vi "FRIC_navX_Internal_USB_ProcessingLoop.vi"(7 "Device Number":T3, 9 "Stream Type":T1=enum."AHRSAndPositioning", 10 "Serial Port":T2=enum."USB 1", 11 "Rate (4Hz-200Hz)":u8=50 min=4 max=200) -> ()   [LabVIEW 2016]
doc: "This navX VI handles the reading/writing for the navX. All of the good stuff is in here.\nTHIS VI SHOULD NOT BE CALLED BY THE USER!"
uses:
  _TypeDefs/Z900_navX_SerialStreamTypeDef.ctl
  _TypeDefs/FRIC_navX_DeviceNumbersTypeDef.ctl
  <vilib>/Rock Robotics/WPI/SerialPort/WPI_SerialPort.ctl
  _TypeDefs/FRIC_navX_I2C Process Loop TypeDef.ctl
  _TypeDefs/FRIC_navX_ProcessingLoopStatesTypeDef_I2C.ctl
  _TypeDefs/Z900_navX_DeviceTypeDef.ctl
  _TypeDefs/Z900_navX_ProtocolTypeDef.ctl
  _TypeDefs/Z900_navX_NotifyPacketTypeDef.ctl
  _TypeDefs/Z900_navX_ActionTypeDef.ctl
  <vilib>/Rock Robotics/SystemInterfaces/i2clib/i2c_bus.ctl
  _TypeDefs/Z900_navX_IntegrationControlRegisters.ctl
  <vilib>/Rock Robotics/WPI/SPI/WPI_SPIDevRef.ctl
  <vilib>/Rock Robotics/SystemInterfaces/spilib/spi_bus.ctl
  <vilib>/Rock Robotics/WPI/SerialPort/WPI_SerialPortRef.ctl
  _Device/_Internal/SERIAL/Z900_navX_SERIAL_ValidatePacketChecksum.vi
  _Device/_Internal/SERIAL/Z900_navX_SERIAL_ValidatePacketTermination.vi
  <vilib>/Rock Robotics/SystemInterfaces/Utilities/FPGA_UtilitiesRead LocalTime.vi
panel:
  in  "Tab Control":enum32{"Page 1", "Page 2"}(tab)
  in  "Halt":bool
  out "Connected 2":bool
  out "Loop Time (ms)":dbl
  out "error":errorcluster
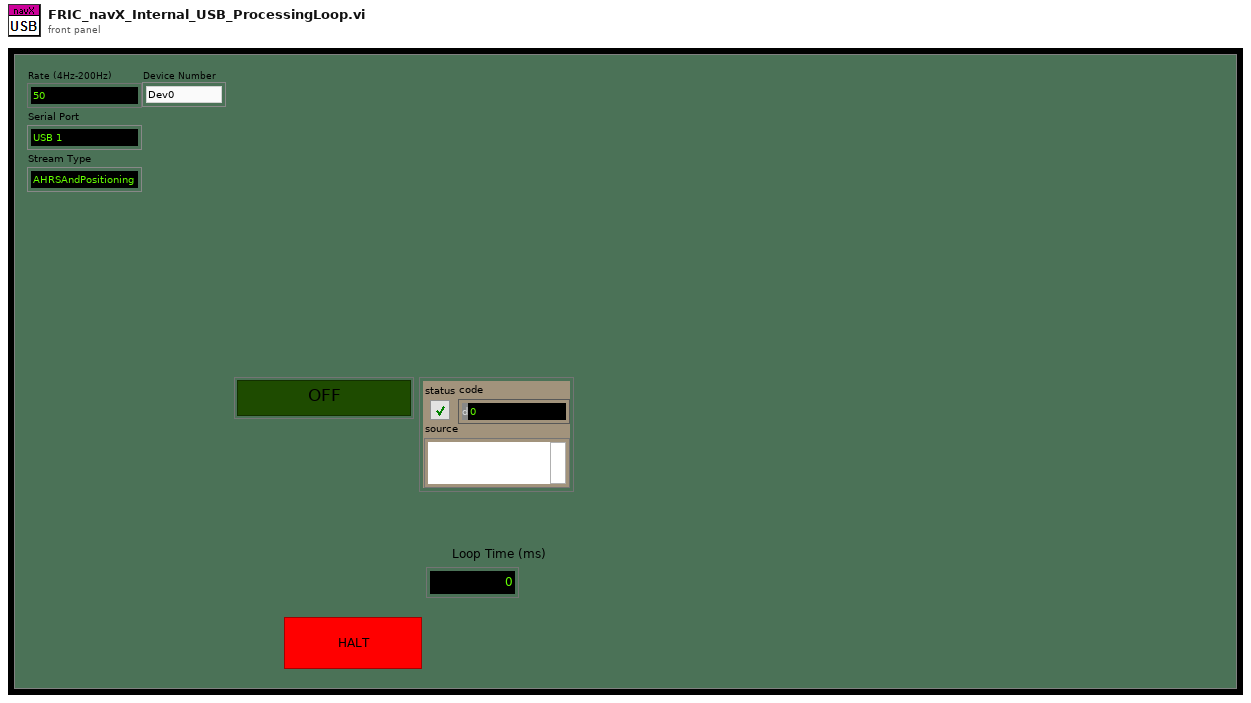
[diagram p1: front panel]
types:
  T1 = typedef "Z900_navX_SerialStreamTypeDef.ctl" = enum16{"YRPH", "Quaterinons", "Gyro/Raw", "AHRS", "AHRSAndPositioning"}
  T2 = typedef "WPI_SerialPort.ctl" = enum16{"Onboard RS-232", "MXP TTL", "USB 1", "USB 2"}
  T3 = typedef "FRIC_navX_DeviceNumbersTypeDef.ctl" = enum16{"Dev0", "Dev1", "Dev2", "Dev3", "Dev4", "Dev5", "Dev6", "Dev7", "Dev8", "Dev9", "Dev10"}
  T4 = typedef "FRIC_navX_I2C Process Loop TypeDef.ctl" = cluster{"State Array":T5[], "error":errorcluster, "FPGA Cluster":cluster{"Last Valid FPGA Time":dbl, "Error Count":i32, "Initialized":bool}, "Device Info":T6, "I2CDevRef":cluster{"DevStatus":errorcluster, "Device Address":u8, "Handle":i32, "I2C Bus":T8}, "Registry":u8[], "Command Array":T9[], "Connected?":bool, "navX Device Memory Size":i32, "notification":T10, "Memory Size Set":bool, "SPIDevRef":T12, "navX Serial Open":cluster{"Stream Type":T1, "Serial Port":T2}, "SerialPortRef":T14, "Serial Read Buffer":string, "Serial Write Buffer":string[], "Device Number":T3, "navX SPI Open":cluster{"SPI Bus":T13, "Clock Rate (Hz)":dbl}}
  T5 = typedef "FRIC_navX_ProcessingLoopStatesTypeDef_I2C.ctl" = enum16{"Process", "INI", "Check Packets Valid", "Close", "Flush Serial", "Generate Command", "Last Packet Valid", "Open", "Read", "Reset Serial", "Set Termination Char", "Update AE", "Wait", "Write", "Exit"}
  T6 = typedef "Z900_navX_DeviceTypeDef.ctl" = cluster{"Interface":cluster{"Protocol":T7, "Update Rate (4Hz-200Hz)":u8, "navX Open TypeDef":variant}, "Notify Packet":refnum<notifier>, "Loop VI Refnum":refnum<vi>, "Ready to Close Occurrence Refnum":refnum<k4>, "Name":string}
  T7 = typedef "Z900_navX_ProtocolTypeDef.ctl" = enum16{"SERIAL", "I2C", "SPI"}
  T8 = typedef "i2c_bus.ctl" = enum16{"I2C On-Board", "I2C MXP", "Invalid"}
  T9 = typedef "Z900_navX_IntegrationControlRegisters.ctl" = u8
  T10 = typedef "Z900_navX_NotifyPacketTypeDef.ctl" = cluster{"navX Action":T11, "Data":variant, "Stream Type":T1, "Device Number":T3}
  T11 = typedef "Z900_navX_ActionTypeDef.ctl" = enum16{"None", "Halt", "Normal Read", "Update Serial Protocol", "Update Rate Htz", "Zero-Yaw", "Zero-Displacement", "Zero-Velocity"}
  T12 = typedef "WPI_SPIDevRef.ctl" = cluster{"DevStatus":errorcluster, "Handle":i32, "SPI Bus":T13}
  T13 = typedef "spi_bus.ctl" = enum16{"SPI On-Board, CS0", "SPI On-Board, CS1", "SPI On-Board, CS2", "SPI On-Board, CS3", "SPI MXP", "Invalid"}
  T14 = typedef "WPI_SerialPortRef.ctl" = cluster{"DevStatus":errorcluster, "Serial Port Name":refnum<visa-resource-name>}
  T15 = cluster{"Last Valid FPGA Time":dbl, "Error Count":i32, "Initialized":bool}
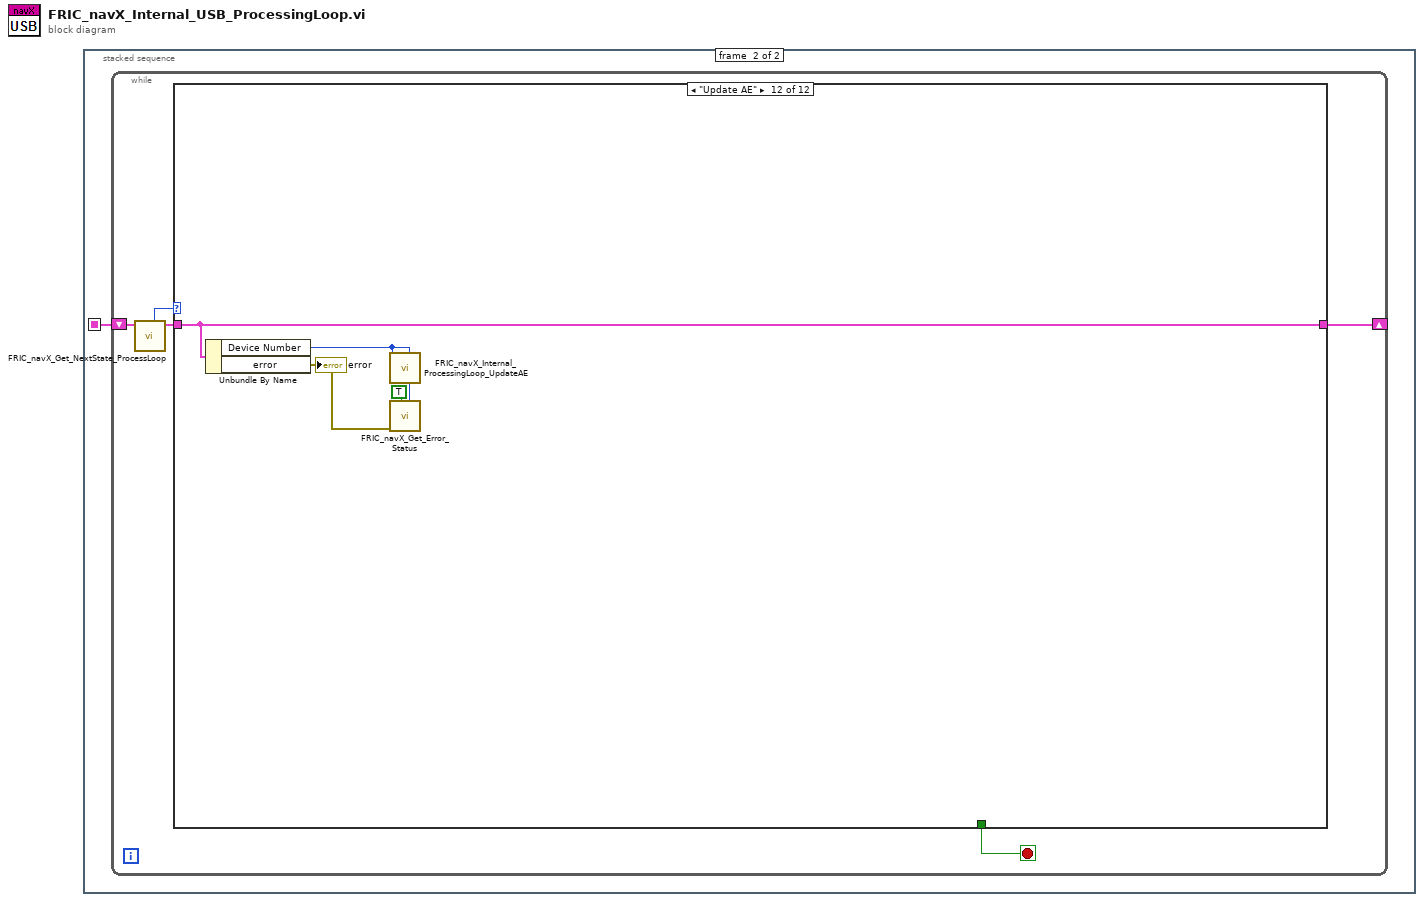
[diagram p0: block diagram]
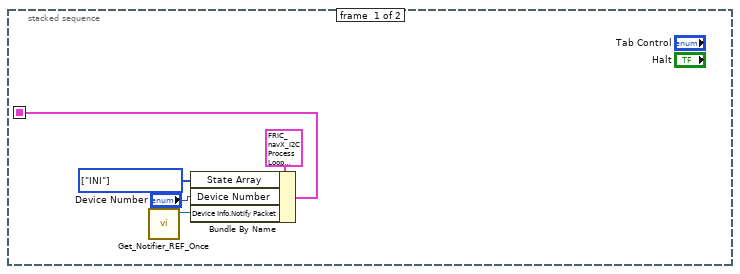
[diagram p2: hidden frame]
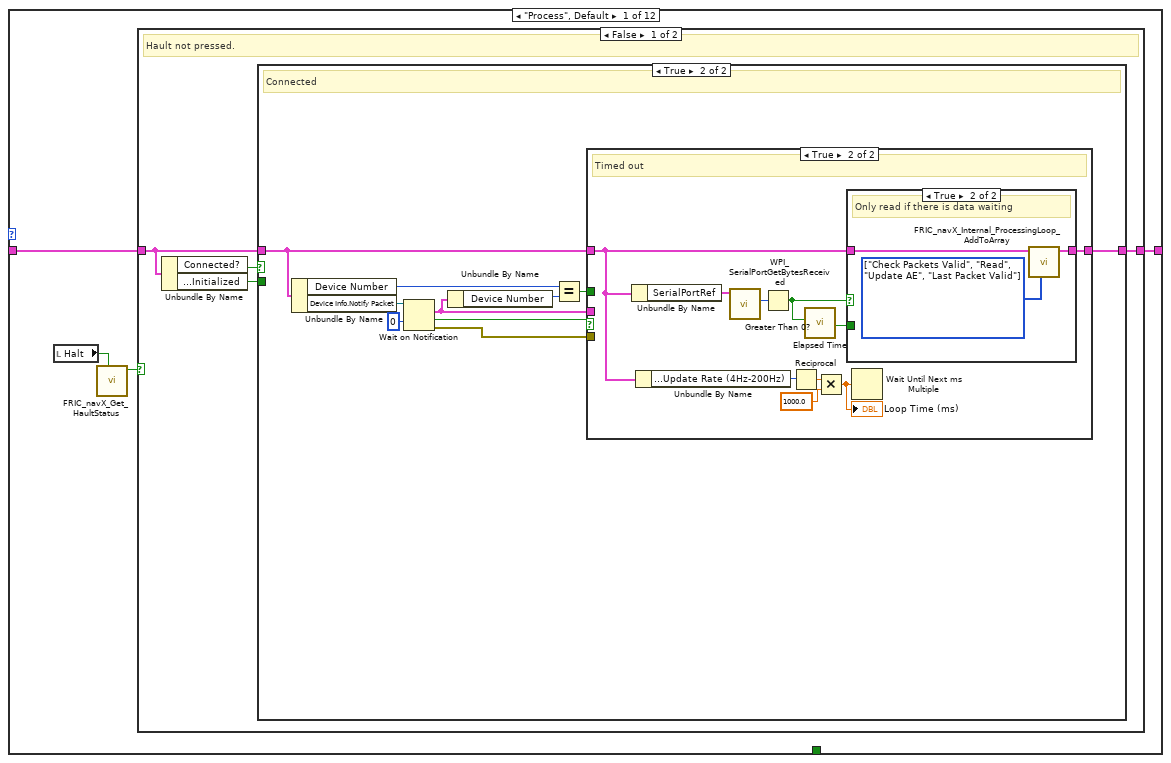
[diagram p3: hidden frame]
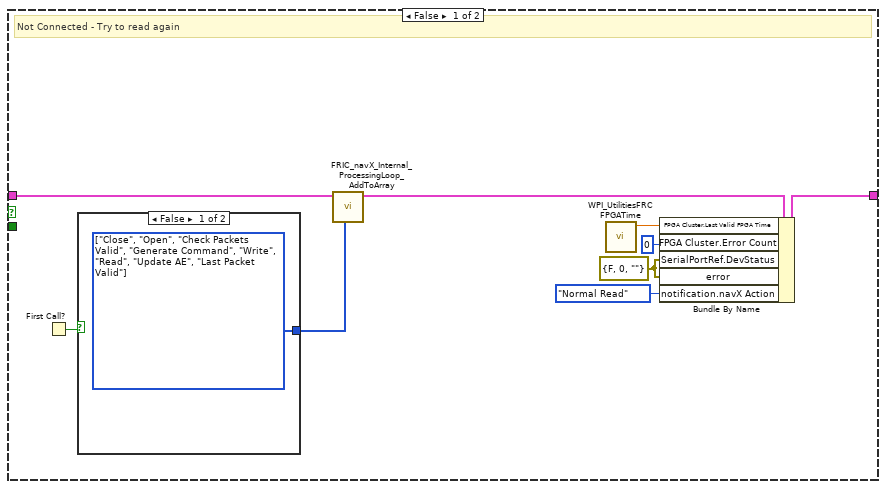
[diagram p4: hidden frame]
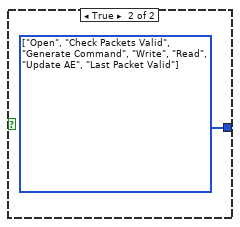
[diagram p5: hidden frame]
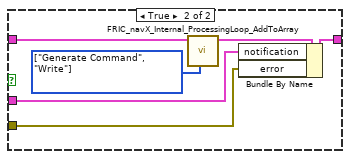
[diagram p7: hidden frame]
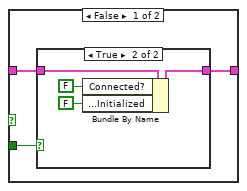
[diagram p8: hidden frame]
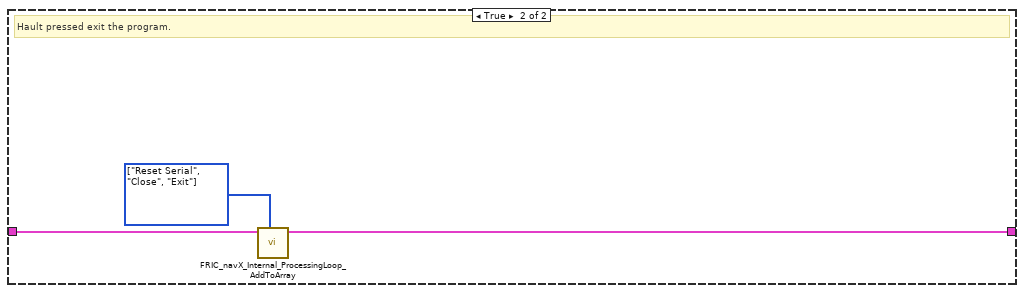
[diagram p10: hidden frame]
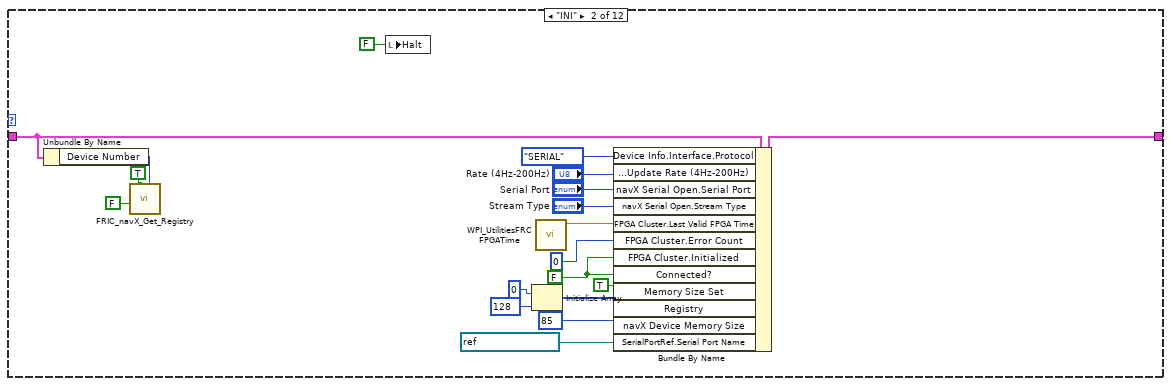
[diagram p11: hidden frame]
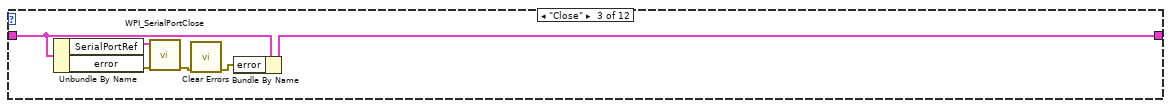
[diagram p12: hidden frame]
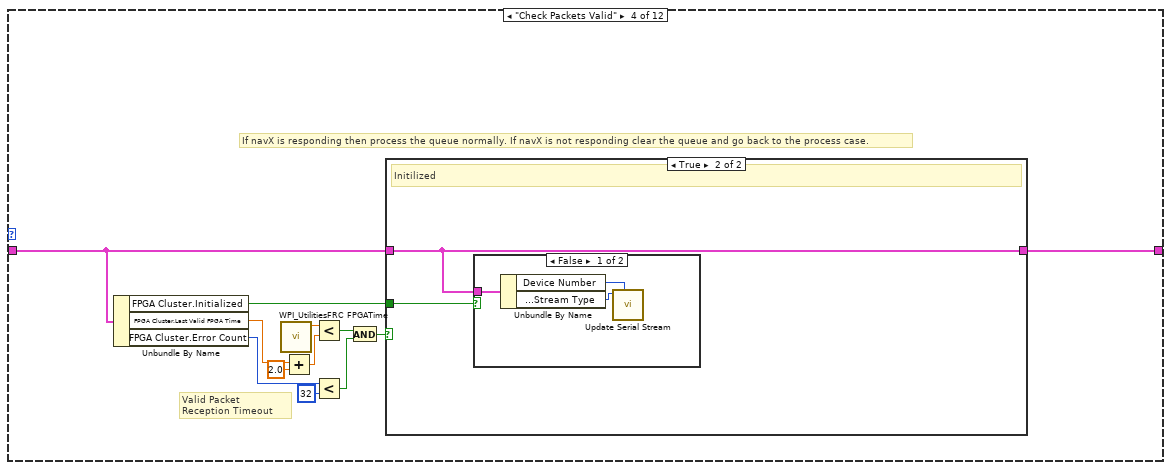
[diagram p13: hidden frame]
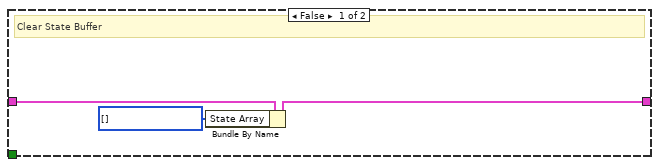
[diagram p14: hidden frame]
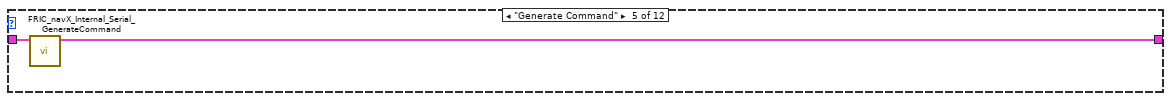
[diagram p16: hidden frame]
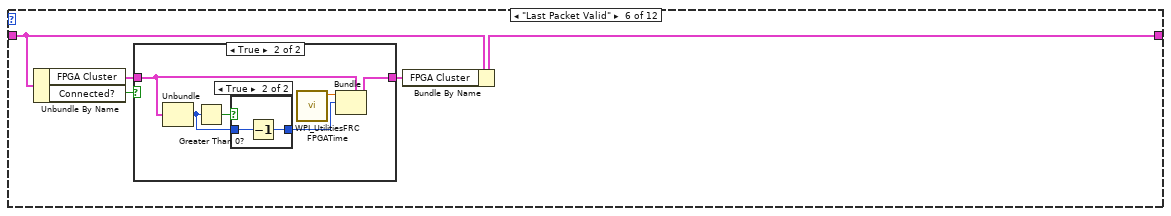
[diagram p17: hidden frame]
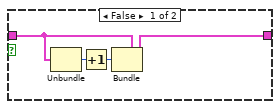
[diagram p18: hidden frame]
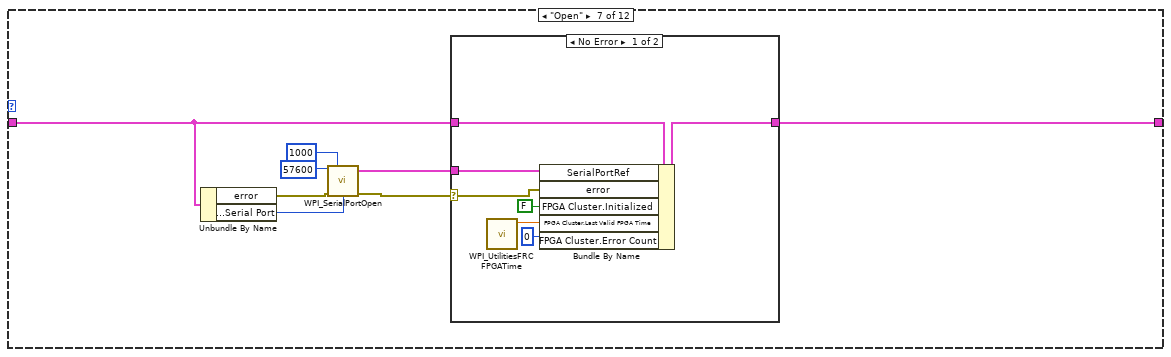
[diagram p20: hidden frame]
diagram:
  n1 = stacked-sequence {
    seq-local: [w5 _] -> [_ w6]
    frame #0 {
      w3 = T5[] [enum."INI"] items=["Process", "INI", "Check Packets Valid", "Close", "Flush Serial", "Generate Command", "Last Packet Valid", "Open", "Read", "Reset Serial", "Set Termination Char", "Update AE", "Wait", "Write", "Exit"] ("State Array")
      n2 = call "Get_Notifier_REF_Once.vi"() -> ("notifier ref out"=w1:refnum<notifier>)  [unwired: 10 in, 1 out]
      n3 = Bundle By Name(cluster=T4 {"State Array"=[enum."INI", enum."Open"], "error"={"status"=FALSE, "code"=0, "source"=""}, "FPGA Cluster"={"Last Valid FPGA Time"=0.0, "Error Count"=0, "Initialized"=FALSE}, "Device Info"={"Interface"={"Protocol"=enum."SERIAL", "Update Rate (4Hz-200Hz)"=4, "navX Open TypeDef"=variant}, "Notify Packet"=refnum, "Loop VI Refnum"=refnum, "Ready to Close Occurrence Refnum"=refnum, "Name"=""}, "I2CDevRef"={"DevStatus"={"status"=FALSE, "code"=0, "source"=""}, "Device Address"=0, "Handle"=0, "I2C Bus"=enum."Invalid"}, "Registry"=[], "Command Array"=[214, 32], "Connected?"=FALSE, "navX Device Memory Size"=85, "notification"={"navX Action"=enum."None", "Data"=variant, "Stream Type"=enum."YRPH", "Device Number"=enum."Dev0"}, "Memory Size Set"=FALSE, "SPIDevRef"={"DevStatus"={"status"=FALSE, "code"=0, "source"=""}, "Handle"=0, "SPI Bus"=enum."SPI On-Board, CS0"}, "navX Serial Open"={"Stream Type"=enum."YRPH", "Serial Port"=enum."Onboard RS-232"}, "SerialPortRef"={"DevStatus"={"status"=FALSE, "code"=0, "source"=""}, "Serial Port Name"=""}, "Serial Read Buffer"="", "Serial Write Buffer"=[], "Device Number"=enum."Dev0", "navX SPI Open"={"SPI Bus"=enum."SPI MXP", "Clock Rate (Hz)"=500000.0}} ("I2C Process Loop TypeDef"), "State Array"=w3, "Device Number"="Device Number", "Device Info.Notify Packet"=w1) -> (w5:T4)
    }
    frame #1 {
      n4 = while {
        shift-right: [w7] -> _
        shift-left: w6 -> [w10]
        stop <- w11 stop-if-true
        n5 = call "FRIC_navX_Get_NextState_ProcessLoop.vi"("I2C Process Loop TypeDef (in)"=w10) -> ("I2C Process Loop TypeDef (out)"=w9:T4, "Current State"=w8:T5)  [unwired: 9 in]
        n6 = case shown="\"Update AE\"" w8 {
          tunnel: [_ _ _ _ _ _ _ _ _ _ TRUE _] -> w11
          tunnel: w9 -> [w14 w82 w101 w106 w123 w127 w149 w176 w194 w207 w214 w224]
          tunnel: [w15 w89 w100 w107 w122 w126 w148 w168 w195 w196 w214 w224] -> w7
          frame "Process", Default {
            n7 = local read "Halt"() -> (w12:bool)
            n8 = call "FRIC_navX_Get_HaultStatus.vi"("Update"=w12) -> ("Hault"=w13:bool)  [unwired: 10 in]
            n9 = case shown="False" w13 {
              tunnel: [w19 w75] -> w15
              tunnel: w14 -> [w17 w76]
              frame False {
                # "Hault not pressed."
                n10 = Unbundle By Name(w17) -> ("Connected?"=w18:bool, "FPGA Cluster.Initialized"=w16:bool)
                n11 = case shown="True" w18 {
                  tunnel: w17 -> [w28 w31]
                  tunnel: [w25 w40] -> w19
                  tunnel: w16 -> [_ _]
                  frame False {
                    w22 = errorcluster {"status"=FALSE, "code"=0, "source"=""} ("SerialPortRef.DevStatus")
                    # "Not Connected - Try to read again"
                    n12 = First Call?() -> (First Call?: T/F=w21:bool)
                    n13 = case shown="False" w21 {
                      tunnel: [w29 w30] -> w27
                      frame False {
                        w29 = T5[] [enum."Close", enum."Open", enum."Check Packets Valid", enum."Generate Command", enum."Write", enum."Read", enum."Update AE", enum."Last Packet Valid"] items=["Process", "INI", "Check Packets Valid", "Close", "Flush Serial", "Generate Command", "Last Packet Valid", "Open", "Read", "Reset Serial", "Set Termination Char", "Update AE", "Wait", "Write", "Exit"]
                      }
                      frame True {
                        w30 = T5[] [enum."Open", enum."Check Packets Valid", enum."Generate Command", enum."Write", enum."Read", enum."Update AE", enum."Last Packet Valid"] items=["Process", "INI", "Check Packets Valid", "Close", "Flush Serial", "Generate Command", "Last Packet Valid", "Open", "Read", "Reset Serial", "Set Termination Char", "Update AE", "Wait", "Write", "Exit"]
                      }
                    }
                    n14 = call "FRIC_navX_Internal_ProcessingLoop_AddToArray.vi"("States Array"=w27, "I2C Process Loop TypeDef (in)"=w28) -> ("I2C Process Loop TypeDef (out)"=w26:T4)  [unwired: 9 in]
                    n15 = call <vilib>:"WPI_UtilitiesFRC FPGATime.vi"() -> ("FPGA Time"=w23:dbl)  [unwired: 10 in, 1 out]
                    n16 = Bundle By Name(cluster=w26, "FPGA Cluster.Last Valid FPGA Time"=w23, "FPGA Cluster.Error Count"=0, "SerialPortRef.DevStatus"=w22, "error"=w22, "notification.navX Action"=Z900_navX_ActionTypeDef."Normal Read") -> (w25:T4)
                  }
                  frame True {
                    # "Connected"
                    n17 = Unbundle By Name(w31) -> ("Device Number"=w34:T3, "Device Info.Notify Packet"=w39:refnum<notifier>)
                    n18 = Wait on Notification(notifier=w39, timeout in ms (-1)=0) -> (notification=w35:T10, timed out?=w36:bool, error out=w37:errorcluster)  [unwired: 2 in, 1 out]
                    n19 = Unbundle By Name(w35) -> ("Device Number"=w33:T3)
                    n20 = Equal?(x=w34, y=w33) -> (x = y?=w32:bool)
                    n21 = case shown="True" w36 {
                      tunnel: w31 -> [w45 w56]
                      tunnel: [w44 w62] -> w40
                      tunnel: w35 -> [w43 _]
                      tunnel: w37 -> [w42 _]
                      tunnel: w32 -> [w41 _]
                      frame False {
                        # "Got a notifier"
                        n22 = case shown="False" w41 {
                          tunnel: w45 -> [w46 w52]
                          tunnel: [w46 w51] -> w44
                          tunnel: w43 -> [_ w50]
                          tunnel: w42 -> [_ w47]
                          frame False {
                          }
                          frame True {
                            w48 = T5[] [enum."Generate Command", enum."Write"] items=["Process", "INI", "Check Packets Valid", "Close", "Flush Serial", "Generate Command", "Last Packet Valid", "Open", "Read", "Reset Serial", "Set Termination Char", "Update AE", "Wait", "Write", "Exit"] ("States Array")
                            n23 = call "FRIC_navX_Internal_ProcessingLoop_AddToArray.vi"("States Array"=w48, "I2C Process Loop TypeDef (in)"=w52) -> ("I2C Process Loop TypeDef (out)"=w49:T4)  [unwired: 9 in]
                            n24 = Bundle By Name(cluster=w49, "notification"=w50, "error"=w47) -> (w51:T4)
                          }
                        }
                      }
                      frame True {
                        # "Timed out"
                        n25 = Unbundle By Name(w56) -> ("SerialPortRef"=w61:T14)
                        n26 = Unbundle By Name(w56) -> ("Device Info.Interface.Update Rate (4Hz-200Hz)"=w57:u8)
                        n27 = call <vilib>:"WPI_SerialPortGetBytesReceived.vi"("SerialPortRef"=w61) -> ("Bytes at Port"=w60:u32)  [unwired: 8 in, 2 out]
                        n28 = Greater Than 0?(x=w60) -> (x > 0?=w55:bool)
                        n29 = Reciprocal(x=w57) -> (1/x=w58:dbl)
                        n30 = call "Elapsed Time"("Reset"=w55) -> ("Time has Elapsed"=w54:bool)  [unwired: 11 in, 7 out]
                        n31 = Multiply(x=w58, y=1000.0) -> (x*y=w53:dbl)
                        "Loop Time (ms)" <- w53
                        n32 = case shown="True" w55 {
                          tunnel: [w64 w72] -> w62
                          tunnel: w56 -> [w65 w71]
                          tunnel: w54 -> [w63 _]
                          frame False {
                            n33 = case shown="True" w63 {
                              tunnel: w65 -> [w66 w70]
                              tunnel: [w66 w69] -> w64
                              frame False {
                              }
                              frame True {
                                n34 = Bundle By Name(cluster=w70, "Connected?"=FALSE, "FPGA Cluster.Initialized"=FALSE) -> (w69:T4)
                              }
                            }
                          }
                          frame True {
                            w73 = T5[] [enum."Check Packets Valid", enum."Read", enum."Update AE", enum."Last Packet Valid"] items=["Process", "INI", "Check Packets Valid", "Close", "Flush Serial", "Generate Command", "Last Packet Valid", "Open", "Read", "Reset Serial", "Set Termination Char", "Update AE", "Wait", "Write", "Exit"]
                            # "Only read if there is data waiting"
                            n35 = call "FRIC_navX_Internal_ProcessingLoop_AddToArray.vi"("States Array"=w73, "I2C Process Loop TypeDef (in)"=w71) -> ("I2C Process Loop TypeDef (out)"=w72:T4)  [unwired: 9 in]
                          }
                        }
                        n36 = Wait Until Next ms Multiple(millisecond multiple=w53) -> ()  [unwired: 1 out]
                      }
                    }
                  }
                }
              }
              frame True {
                w74 = T5[] [enum."Reset Serial", enum."Close", enum."Exit"] items=["Process", "INI", "Check Packets Valid", "Close", "Flush Serial", "Generate Command", "Last Packet Valid", "Open", "Read", "Reset Serial", "Set Termination Char", "Update AE", "Wait", "Write", "Exit"] ("States Array")
                # "Hault pressed exit the program."
                n37 = call "FRIC_navX_Internal_ProcessingLoop_AddToArray.vi"("States Array"=w74, "I2C Process Loop TypeDef (in)"=w76) -> ("I2C Process Loop TypeDef (out)"=w75:T4)  [unwired: 9 in]
              }
            }
          }
          frame "INI" {
            w87 = FALSE ("Initialized")
            n38 = Unbundle By Name(w82) -> ("Device Number"=w81:T3)
            n39 = call "FRIC_navX_Get_Registry.vi"("Device Number"=w81, "Update"=TRUE, "Connected?"=FALSE) -> ()  [unwired: 7 in, 2 out]
            n40 = local write "Halt"(FALSE ("Halt")) -> ()
            n41 = Initialize Array(u8 0 ("Received Data"), 128 ("hex")) -> (w85:u8[])
            n42 = call <vilib>:"WPI_UtilitiesFRC FPGATime.vi"() -> ("FPGA Time"=w91:dbl)  [unwired: 10 in, 1 out]
            n43 = Bundle By Name(cluster=w82, "Device Info.Interface.Protocol"=Z900_navX_ProtocolTypeDef."SERIAL" ("Protocol"), "Device Info.Interface.Update Rate (4Hz-200Hz)"="Rate (4Hz-200Hz)", "navX Serial Open.Serial Port"="Serial Port", "navX Serial Open.Stream Type"="Stream Type", "FPGA Cluster.Last Valid FPGA Time"=w91, "FPGA Cluster.Error Count"=0 ("Error Count"), "FPGA Cluster.Initialized"=w87, "Connected?"=w87, "Memory Size Set"=TRUE, "Registry"=w85, "navX Device Memory Size"=85 ("hex"), "SerialPortRef.Serial Port Name"=refnum<visa-resource-name> "ASRL3::INSTR" ("Serial Port Name")) -> (w89:T4)
          }
          frame "Close" {
            n44 = Unbundle By Name(w101) -> ("SerialPortRef"=w98:T14, "error"=w97:errorcluster)
            n45 = call <vilib>:"WPI_SerialPortClose.vi"("error in (no error)"=w97, "SerialPortRef"=w98) -> ("error out"=w96:errorcluster)  [unwired: 9 in]
            n46 = call <vilib>:"Clear Errors.vi"("error in (no error)"=w96) -> ("error out"=w99:errorcluster)  [unwired: 5 in, 1 out]
            n47 = Bundle By Name(cluster=w101, "error"=w99) -> (w100:T4)
          }
          frame "Check Packets Valid" {
            # "If navX is responding then process the queue normally. If navX is not responding clear the queue and go back to the process case."
            # "Valid Packet Reception Timeout"
            n48 = Unbundle By Name(w106) -> ("FPGA Cluster.Initialized"=w102:bool, "FPGA Cluster.Last Valid FPGA Time"=w105:dbl, "FPGA Cluster.Error Count"=w104:i32)
            n49 = call <vilib>:"WPI_UtilitiesFRC FPGATime.vi"() -> ("FPGA Time"=w111:dbl)  [unwired: 10 in, 1 out]
            n50 = Add(x=w105, y=2.0) -> (x+y=w112:dbl)
            n51 = Less?(x=w111, y=w112) -> (x < y?=w109:bool)
            n52 = Less?(x=w104, y=32) -> (x < y?=w108:bool)
            n53 = And(x=w109, y=w108) -> (x .and. y?=w103:bool)
            n54 = case shown="True" w103 {
              tunnel: w106 -> [w116 w118]
              tunnel: [w115 w118] -> w107
              tunnel: w102 -> [_ w117]
              frame False {
                w114 = T5[] [] items=["Process", "INI", "Check Packets Valid", "Close", "Flush Serial", "Generate Command", "Last Packet Valid", "Open", "Read", "Reset Serial", "Set Termination Char", "Update AE", "Wait", "Write", "Exit"] ("f")
                # "Clear State Buffer"
                n55 = Bundle By Name(cluster=w116, "State Array"=w114) -> (w115:T4)
              }
              frame True {
                # "Initilized"
                n56 = case shown="False" w117 {
                  tunnel: w118 -> [w119 _]
                  frame False {
                    n57 = Unbundle By Name(w119) -> ("Device Number"=w120:T3, "navX Serial Open.Stream Type"=w121:T1)
                    n58 = call "Update Serial Stream.vi"("Device Number"=w120, "Stream Type"=w121) -> ()  [unwired: 10 in]
                  }
                  frame True {
                  }
                }
              }
            }
          }
          frame "Generate Command" {
            n59 = call "FRIC_navX_Internal_Serial_GenerateCommand.vi"("Serial Process Loop TypeDef (in)"=w123) -> ("Serial Process Loop TypeDef (out)"=w122:T4)  [unwired: 10 in]
          }
          frame "Last Packet Valid" {
            n60 = Unbundle By Name(w127) -> ("FPGA Cluster"=w128:T15, "Connected?"=w124:bool)
            n61 = case shown="True" w124 {
              tunnel: [w131 w138] -> w125
              tunnel: w128 -> [w130 w134]
              frame False {
                n62 = Unbundle(w130) -> ("Error Count"=w129:i32)  [unwired: 2 out]
                n63 = Increment(x=w129) -> (x+1=w132:i32)
                n64 = Bundle(cluster=w130, "Error Count"=w132) -> (w131:T15)  [unwired: 2 in]
              }
              frame True {
                n65 = Unbundle(w134) -> ("Error Count"=w133:i32)  [unwired: 2 out]
                n66 = Greater Than 0?(x=w133) -> (x > 0?=w136:bool)
                n67 = case shown="True" w136 {
                  tunnel: [w139 w141] -> w135
                  tunnel: w133 -> [w139 w140]
                  frame False {
                  }
                  frame True {
                    n68 = Decrement(x=w140) -> (x-1=w141:i32)
                  }
                }
                n69 = call <vilib>:"WPI_UtilitiesFRC FPGATime.vi"() -> ("FPGA Time"=w137:dbl)  [unwired: 10 in, 1 out]
                n70 = Bundle(cluster=w134, "Last Valid FPGA Time"=w137, "Error Count"=w135) -> (w138:T15)  [unwired: 1 in]
              }
            }
            n71 = Bundle By Name(cluster=w127, "FPGA Cluster"=w125) -> (w126:T4)
          }
          frame "Open" {
            n72 = Unbundle By Name(w149) -> ("error"=w145:errorcluster, "navX Serial Open.Serial Port"=w142:T2)
            n73 = call <vilib>:"WPI_SerialPortOpen.vi"("Baud Rate"=u32 57600, "Timeout Value (ms)"=u32 1000, "error in (no error)"=w145, "Serial Port"=w142) -> ("SerialPortRef"=w147:T14, "error out"=w146:errorcluster)  [unwired: 10 in]
            n74 = case shown="No Error" w146 {
              selector: w146 -> [w150 _]
              tunnel: w149 -> [w156 w159]
              tunnel: [w155 w158] -> w148
              tunnel: w147 -> [w153 _]
              frame No Error {
                n75 = call <vilib>:"WPI_UtilitiesFRC FPGATime.vi"() -> ("FPGA Time"=w152:dbl)  [unwired: 10 in, 1 out]
                n76 = Bundle By Name(cluster=w156, "SerialPortRef"=w153, "error"=w150, "FPGA Cluster.Initialized"=FALSE ("Initialized"), "FPGA Cluster.Last Valid FPGA Time"=w152, "FPGA Cluster.Error Count"=0) -> (w155:T4)
              }
              frame Error {
                w157 = T5[] [] items=["Process", "INI", "Check Packets Valid", "Close", "Flush Serial", "Generate Command", "Last Packet Valid", "Open", "Read", "Reset Serial", "Set Termination Char", "Update AE", "Wait", "Write", "Exit"] ("State Array")
                # "Clear State Array on Error"
                n77 = Bundle By Name(cluster=w159, "State Array"=w157) -> (w158:T4)
              }
            }
          }
          frame "Read" {
            # "I look to see how many bytes are waiting at the serial port. If there is more that 128 I send 128 read and then tell the loop to read again. If there is less than 128 I read what is left and tell the loop to decode the buffer."
            n78 = Unbundle By Name(w176) -> ("Serial Read Buffer"=w181:string, "SerialPortRef"=w182:T14, "SerialPortRef.Serial Port Name"=w184:refnum<visa-resource-name>, "error"=w183:errorcluster, "Device Number"=w160:T3, "Registry"=w177:u8[])
            n79 = property class="Instr"(reference=w184, error in=w183) -> (error out=w178:errorcluster, "Bytes at Port"=w164:u32)  [unwired: 1 in]
            n80 = Greater?(x=w164, y=u32 128) -> (0:w167:bool)
            n81 = Select(t=u32 128 ("y"), s=w167, f=w164) -> (s? t:f=w163:u32)
            n82 = call <vilib>:"WPI_SerialPortRead.vi"("error in (no error)"=w178, "Num Bytes to Read"=w163, "SerialPortRef"=w182) -> ("error out"=w165:errorcluster, "Buffer"=w175:string)  [unwired: 6 in, 1 out]
            n83 = Concatenate Strings(w181, w175) -> (w174:string)
            n84 = Not(x=w165) -> (.not. x?=w166:bool)
            "Connected 2" <- w166
            n85 = call "Z900_navX_SERIAL_CapturePacket.vi"("Buffer"=w174) -> ("Packet"=w171:string, "Buffer"=w173:string)  [unwired: 7 in, 2 out]
            n86 = call "Z900_navX_SERIAL_DecodePacket.vi"("Data (in)"=w177, "Packet (in)"=w171) -> ("empty?"=w162:bool, "Data"=w172:u8[])  [unwired: 6 in, 2 out]
            n87 = Not(x=w162) -> (.not. x?=w161:bool)
            n88 = call "FRIC_navX_Get_Registry.vi"("Device Number"=w160, "Update"=w161, "Connected?"=w166, "Registry (in)"=w172) -> ()  [unwired: 6 in, 2 out]
            n89 = Bundle By Name(cluster=w176, "Serial Read Buffer"=w173, "Connected?"=w166, "error"=w165) -> (w169:T4)
            n90 = call "FRIC_navX_Get_Connect_Status.vi"("Device Number"=w160, "Update"=TRUE, "Connected"=w166) -> ()  [unwired: 8 in, 1 out]
            n91 = case shown="False" w167 {
              tunnel: w169 -> [w185 w189]
              tunnel: [w185 w188] -> w168
              frame False {
              }
              frame True {
                w187 = T5[] [enum."Read"] items=["Process", "INI", "Check Packets Valid", "Close", "Flush Serial", "Generate Command", "Last Packet Valid", "Open", "Read", "Reset Serial", "Set Termination Char", "Update AE", "Wait", "Write", "Exit"] ("States Array")
                n92 = call "FRIC_navX_Internal_ProcessingLoop_AddToArray.vi"("Add to beginning"=TRUE, "States Array"=w187, "I2C Process Loop TypeDef (in)"=w189) -> ("I2C Process Loop TypeDef (out)"=w188:T4)  [unwired: 8 in]
              }
            }
          }
          frame "Reset Serial" {
            n93 = Unbundle By Name(w194) -> ("SerialPortRef"=w193:T14, "error"=w191:errorcluster)
            n94 = call <vilib>:"WPI_SerialPortReset.vi"("error in (no error)"=w191, "SerialPortRef"=w193) -> ("error out"=w190:errorcluster, "SerialPortRef"=w192:T14)  [unwired: 8 in]
            n95 = Bundle By Name(cluster=w194, "SerialPortRef"=w192, "error"=w190) -> (w195:T4)
          }
          frame "Write" {
            n96 = Unbundle By Name(w207) -> ("SerialPortRef"=w205:T14, "Serial Write Buffer"=w202:string[], "SerialPortRef.DevStatus"=w206:errorcluster)
            n97 = Delete From Array(array=w202, index=0) -> (deleted portion=w201:string, array with subset deleted=w198:string[])  [unwired: 1 in]
            n98 = call <vilib>:"WPI_SerialPortWrite.vi"("error in (no error)"=w206, "Buffer"=w201, "SerialPortRef"=w205) -> ("error out"=w204:errorcluster, "SerialPortRef"=w203:T14)  [unwired: 6 in, 1 out]
            n99 = Empty Array?(array=w198) -> (empty?=w197:bool)
            n100 = Bundle By Name(cluster=w207, "SerialPortRef"=w203, "error"=w204, "Serial Write Buffer"=w198) -> (w199:T4)
            n101 = case shown="True" w197 {
              tunnel: [w211 w212] -> w196
              tunnel: w199 -> [w210 w212]
              frame False {
                w209 = T5[] [enum."Write"] items=["Process", "INI", "Check Packets Valid", "Close", "Flush Serial", "Generate Command", "Last Packet Valid", "Open", "Read", "Reset Serial", "Set Termination Char", "Update AE", "Wait", "Write", "Exit"] ("States Array")
                # "Write again because buffer is not empty."
                n102 = call "FRIC_navX_Internal_ProcessingLoop_AddToArray.vi"("Add to beginning"=TRUE, "States Array"=w209, "I2C Process Loop TypeDef (in)"=w210) -> ("I2C Process Loop TypeDef (out)"=w211:T4)  [unwired: 8 in]
              }
              frame True {
                # "Process the rest of the state array"
              }
            }
          }
          frame "Exit" {
            n103 = Unbundle By Name(w214) -> ("Device Info"=w213:T6)
            n104 = in-place {
              in-place-border: [TRUE] -> w216
              in-place-border: w213 -> [w218]
              # "Set Occurence of Close"
              n105 = Unbundle By Name(w218) -> ("Ready to Close Occurrence Refnum"=w220:refnum<k4>)
              n106 = local write "Halt"(FALSE ("Halt")) -> ()
              n107 = Set Occurrence(w220) -> ()
            }
            n108 = Stop(stop? (T)=w216) -> ()
          }
          frame "Update AE" {
            n109 = Unbundle By Name(w224) -> ("Device Number"=w221:T3, "error"=w223:errorcluster)
            "error" <- w223
            n110 = call "FRIC_navX_Internal_ProcessingLoop_UpdateAE.vi"("Device Number"=w221) -> ()  [unwired: 15 in]
            n111 = call "FRIC_navX_Get_Error_Status.vi"("Device Number"=w221, "Update"=TRUE, "error in"=w223) -> ()  [unwired: 8 in, 1 out]
          }
        }
      }
    }
  }
